vi "TSE_Wait_For_Init.vi"() -> (0 "error IO":errorcluster, 2 "Aborted":bool)   [LabVIEW 2014]
uses:
  CustomControls/TSE_Status.ctl
  CustomControls/Program_States.ctl
panel:
  out "TSE Status":T1={"Return Code"=0, "Message"="", "error in (no error)"={"status"=FALSE, "code"=0, "source"=""}, "Program State"=enum."Ön Yükleme Tamam", "Test A. Suresi"=0}
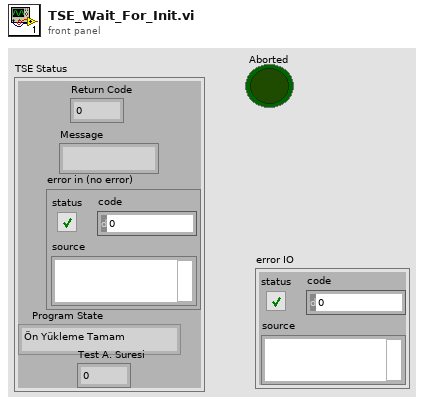
[diagram p1: front panel]
types:
  T1 = typedef "TSE_Status.ctl" = cluster{"Return Code":i32, "Message":string, "error in (no error)":errorcluster, "Program State":T2, "Test A. Suresi":u32}
  T2 = typedef "Program_States.ctl" = enum16{"Ön Yükleme", "TSE Baslat", "Kalibratöre Baglan", "Kalibratörü Baslat", "Ön Yükleme Tamam", "Frekans Testi", "Gerilim Testi", "Akim Testi", "Aktif Guc Testi", "Reaktif Guc Testi", "AC Akim Harmonik Testi", "AC Gerilim Harmonik Testi", "Flicker Testi", "Rapor Cikarma", "Yeniden Başlat", "Bekleme", "Durdur"}
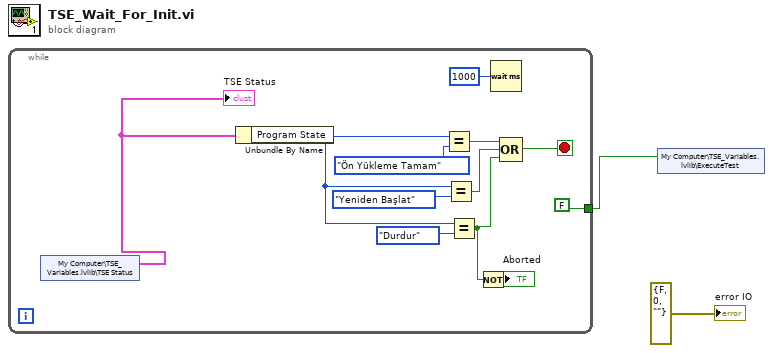
[diagram p0: block diagram]
diagram:
  n1 = while {
    tunnel: [FALSE ("ExecuteTest")] -> w1
    stop <- w13 stop-if-true
    n2 = shared-variable "My Computer\\TSE_Variables.lvlib\\TSE Status"() -> (w3:T1)  [unwired: 1 in, 1 out]
    "TSE Status" <- w3
    n3 = Unbundle By Name(w3) -> ("Program State"=w7:T2)
    n4 = Equal?(x=w7, y=Program_States."Ön Yükleme Tamam" ("Ring")) -> (x = y?=w12:bool)
    n5 = Equal?(x=w7, y=Program_States."Yeniden Başlat" ("Ring")) -> (x = y?=w11:bool)
    n6 = Equal?(x=w7, y=Program_States."Durdur") -> (x = y?=w8:bool)
    n7 = Not(x=w8) -> (.not. x?=→"Aborted":bool)
    n8 = Wait (ms)(milliseconds to wait=u32 1000) -> ()  [unwired: 1 out]
    n9 = Compound Arithmetic op=OR(w12, w11, w8) -> (w13:bool)
  }
  n10 = shared-variable "My Computer\\TSE_Variables.lvlib\\ExecuteTest"(w1) -> ()  [unwired: 1 in, 1 out]
  "error IO" <- errorcluster {"status"=FALSE, "code"=0, "source"=""} ("error IO")
